vi "PZT steporslide.vi"(2 "error in (no error)":errorcluster caption="错误输入（无错误）", 3 "运行模式":u16(ring) items=["Step", "Slide"], 4 "VISA resource name":refnum<visa-resource-name> caption="VISA资源名称") -> (0 "错误输出":errorcluster, 1 "VISA资源名称输出":refnum<visa-resource-name>)   [LabVIEW 2019]
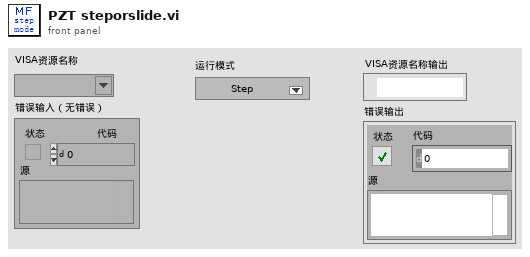
[diagram p1: front panel]
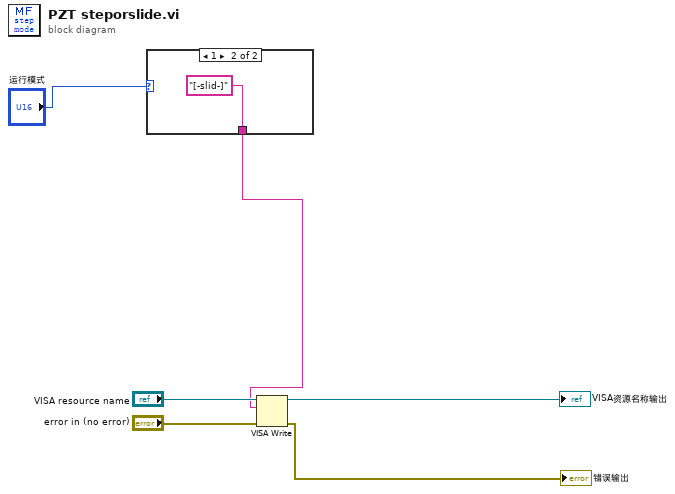
[diagram p0: block diagram]
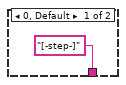
[diagram p2: hidden frame]
diagram:
  n1 = case shown="1" "运行模式" {
    tunnel: ["[-step-]" ("字符串") "[-slid-]" ("字符串")] -> w2
    frame 0, Default {
    }
    frame 1 {
    }
  }
  n2 = VISA Write(VISA resource name="VISA resource name", write buffer=w2, error in (no error)="error in (no error)") -> (VISA resource name out=→"VISA资源名称输出":refnum<visa-resource-name>, error out=→"错误输出":errorcluster)  [unwired: 1 out]
